vi "Test_Draw_Text_ARGB.vi"(8 "error in (no error)":errorcluster, 11 "Test Case In":refnum<class "Image.lvclass">) -> (0 "error out":errorcluster, 3 "Test Case Out":refnum<class "Image.lvclass">)   [LabVIEW 2020, in "g_ar_toolkit.test.lvlib" / "Image.lvclass"]
uses:
  Image.lvclass
  Image.lvclass/Image.ctl
  g_ar_toolkit.image/g_ar_toolkit.image.lvlib
  g_ar_toolkit.image/CreateEmptyImageARGB.vi
  g_ar_toolkit.image/ARGB Colour.ctl
  g_ar_toolkit.image/Image Size (Fixed).ctl
  g_ar_toolkit.image/Image Point (Fixed).ctl
  g_ar_toolkit.image/Line Type.ctl
  g_ar_toolkit.image/Font Face.ctl
  g_ar_toolkit.image/Text Drawing Settings.ctl
  4993e8ee-a06a-463a-9684-69129f64d5ce.vi
panel:
  out "Picture":picture
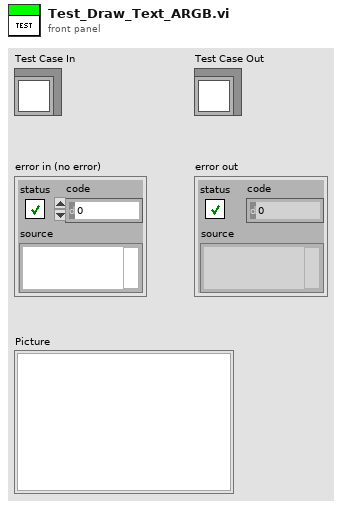
[diagram p1: front panel]
types:
  T1 = typedef "g_ar_toolkit.image.lvlib/Text Drawing Settings.ctl" = cluster{"OpenCV Font Face":T2, "Font Scale":dbl}
  T2 = typedef "g_ar_toolkit.image.lvlib/Font Face.ctl" = enum16{"FONT_HERSHEY_SIMPLEX", "FONT_HERSHEY_PLAIN", "FONT_HERSHEY_DUPLEX", "FONT_HERSHEY_COMPLEX", "FONT_HERSHEY_TRIPLEX", "FONT_HERSHEY_COMPLEX_SMALL", "FONT_HERSHEY_SCRIPT_SIMPLEX", "FONT_HERSHEY_SCRIPT_COMPLEX", "FONT_ITALIC"}
  T3 = typedef "g_ar_toolkit.image.lvlib/Line Type.ctl" = enum8{"FILLED", "LINE_4", "LINE_8", "LINE_AA"}
  T4 = typedef "g_ar_toolkit.image.lvlib/ARGB Colour.ctl" = cluster{"Alpha":u8, "RGB":u32}
  T5 = typedef "g_ar_toolkit.image.lvlib/Image Point (Fixed).ctl" = cluster{"x":i32, "y":i32}
  T6 = typedef "g_ar_toolkit.image.lvlib/Image Size (Fixed).ctl" = cluster{"Width":u16, "Height":u16}
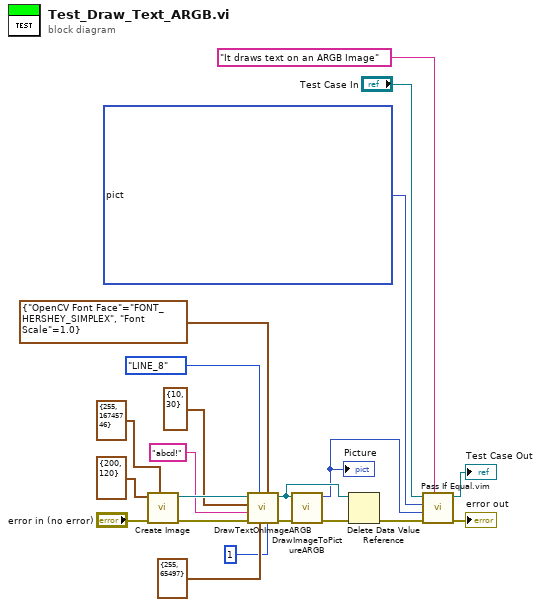
[diagram p0: block diagram]
diagram:
  n1 = call-poly "Create Image.vi"("Colour (Default: Black)"=T4 {"Alpha"=255, "RGB"=16745746}, "error in (no error)"="error in (no error)", "Preallocated Image Size (Default: 0,0)"=T6 {"Width"=200, "Height"=120}) -> ("error out"=w14:errorcluster, "New ARGB Image"=w15:refnum<data-value>)  [unwired: 7 in]
  n2 = call "DrawTextOnImageARGB.vi"("Thickness (Default: 1)"=u16 1, "Text Drawing Settings (Default: Simplex)"=T1 {"OpenCV Font Face"=enum."FONT_HERSHEY_SIMPLEX", "Font Scale"=1.0} ("Text Drawing Settings (Default: Simplex, Top-Left)"), "ARGB Colour"=T4 {"Alpha"=255, "RGB"=65497}, "OpenCV Line Type (Default LINE_8)"=Line_Type."LINE_8", "error in (no error)"=w14, "Text"="abcd!", "Origin"=T5 {"x"=10, "y"=30} ("Centre"), "ARGB Image"=w15) -> ("error out"=w12:errorcluster, "ARGB Image (Duplicate)"=w13:refnum<data-value>)  [unwired: 2 in]
  n3 = call "DrawImageToPictureARGB.vi"("error in (no error)"=w12, "ARGB Image Source"=w13) -> ("error out"=w11:errorcluster, "Picture"=w5:picture)  [unwired: 8 in]
  "Picture" <- w5
  n4 = Delete Data Value Reference(data value reference=w13, error in=w11) -> (error out=w17:errorcluster)  [unwired: 1 out]
  n5 = call "Pass If Equal.vim"("Description"="It draws text on an ARGB Image", "error in (no error)"=w17, "Actual"=w5, "Expected"=picture bytes[72030] ("Picture"), "LUnit Test Case In"="Test Case In") -> ("error out"=→"error out":errorcluster, "LUnit Test Case Out"=→"Test Case Out":refnum<class "Image.lvclass">)  [unwired: 5 in]
